vi "Const_ADO.vi"() -> (0 "ADOMapper":refnum<class "ADOMapper.lvclass">)   [LabVIEW 2020]
uses:
  <vilib>/Viviota/shared/ORM_ADONet.lvlibp
  <vilib>/Viviota/shared/ORM_ADONet.lvlibp/ADOMapper/ADOMapper.lvclass
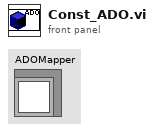
[diagram p1: front panel]
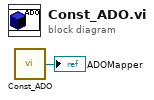
[diagram p0: block diagram]
diagram:
  n1 = call <vilib>:"Const_ADO.vi"() -> ("ADOMapper"=→"ADOMapper":refnum<class "ADOMapper.lvclass">)
